vi "ocr subvi22.vi"(7 "char set file path":path, 9 "Manual ROI selection":bool, 10 "Image":T3) -> (1 "Read String":string, 3 "Image 2":T3(plugin-control))   [LabVIEW 2011]
uses:
  <vilib>/vision/NI_Vision_Development_Module.lvlib
  <vilib>/vision/Image Controls.llb/IMAQ Image.ctl
  <vilib>/vision/OCR.llb/IMAQ OCR Character Report 2.ctl
panel:
  out "subarray":i32[](array[numeric])
  out "Coordinates":i32[][](array[numeric])
  out "ROI Bounding Characters":T1 {"Contours"."Type" items=["No Selection", "Point", "Line", "Rectangle", "Oval", "Polygon", "Free", "Annulus", "Unused2", "Unused3", "Broken Line", "Free Hand Line", "Rotated Rectangle"]}
  out "Global Rectangle":i32[](array[numeric])
  out "Character Reports":T2[](array[typedef]) {"Character Statistics"."Threshold Range"."Upper value" format="%.2f"; "Character Statistics"."Threshold Range"."Lower value" format="%.2f"}
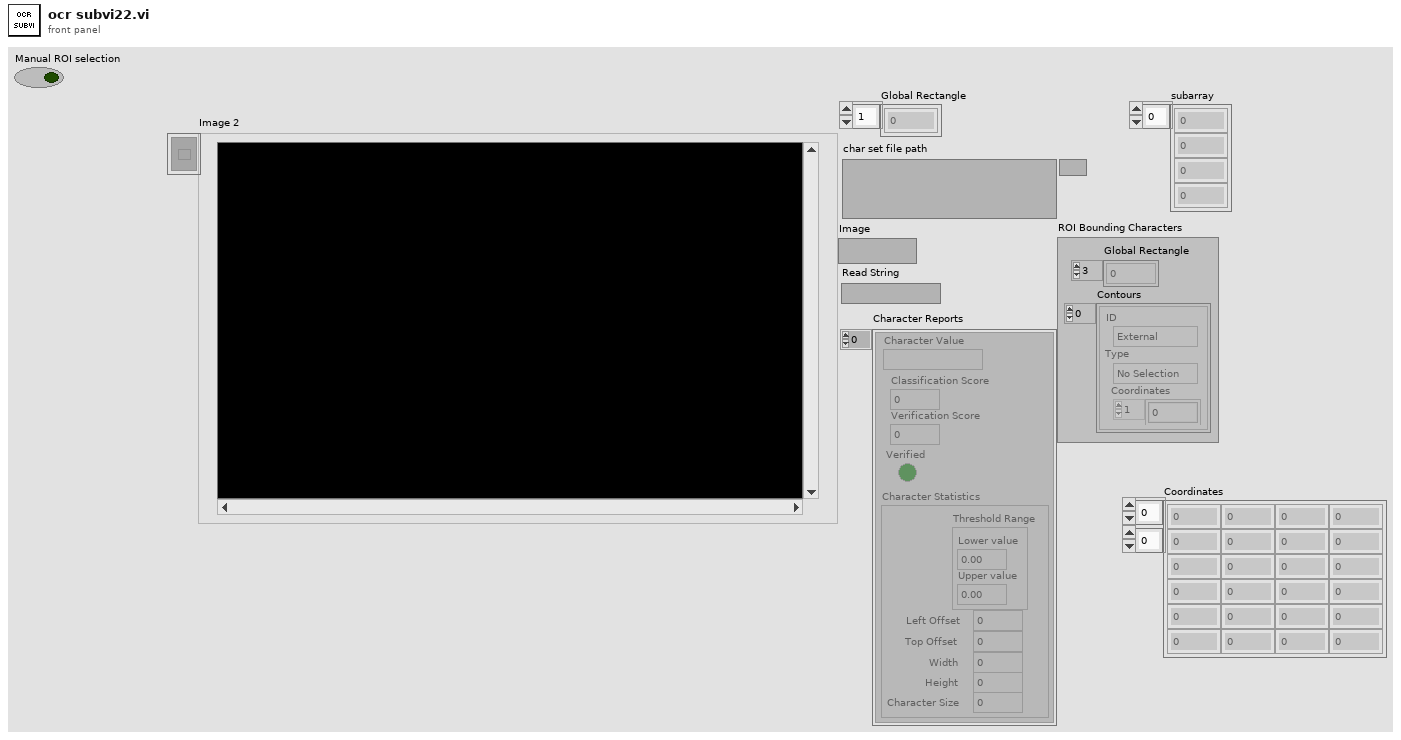
[diagram p1: front panel]
types:
  T1 = cluster{"Global Rectangle":i32[], "Contours":cluster{"ID":enum32{"External", "Internal"}, "Type":u32, "Coordinates":i32[]}[]}
  T2 = typedef "IMAQ OCR Character Report 2.ctl" = cluster{"Character Value":string, "Classification Score":i32, "Verification Score":i32, "Verified":bool, "Character Statistics":cluster{"Threshold Range":cluster{"Lower value":sgl, "Upper value":sgl}, "Left Offset":i32, "Top Offset":i32, "Width":i32, "Height":i32, "Character Size":i32}}
  T3 = typedef "IMAQ Image.ctl" = refnum<image>
  T4 = typedef "IMAQ OCR Session.ctl" = refnum<k1>
  T5 = cluster{i32[], cluster{"Contour Type":u32, "ROI Type":u32, i32[]}[]}
  T6 = cluster{"ID":enum32{"External", "Internal"}, "Type":u32, "Coordinates":i32[]}[]
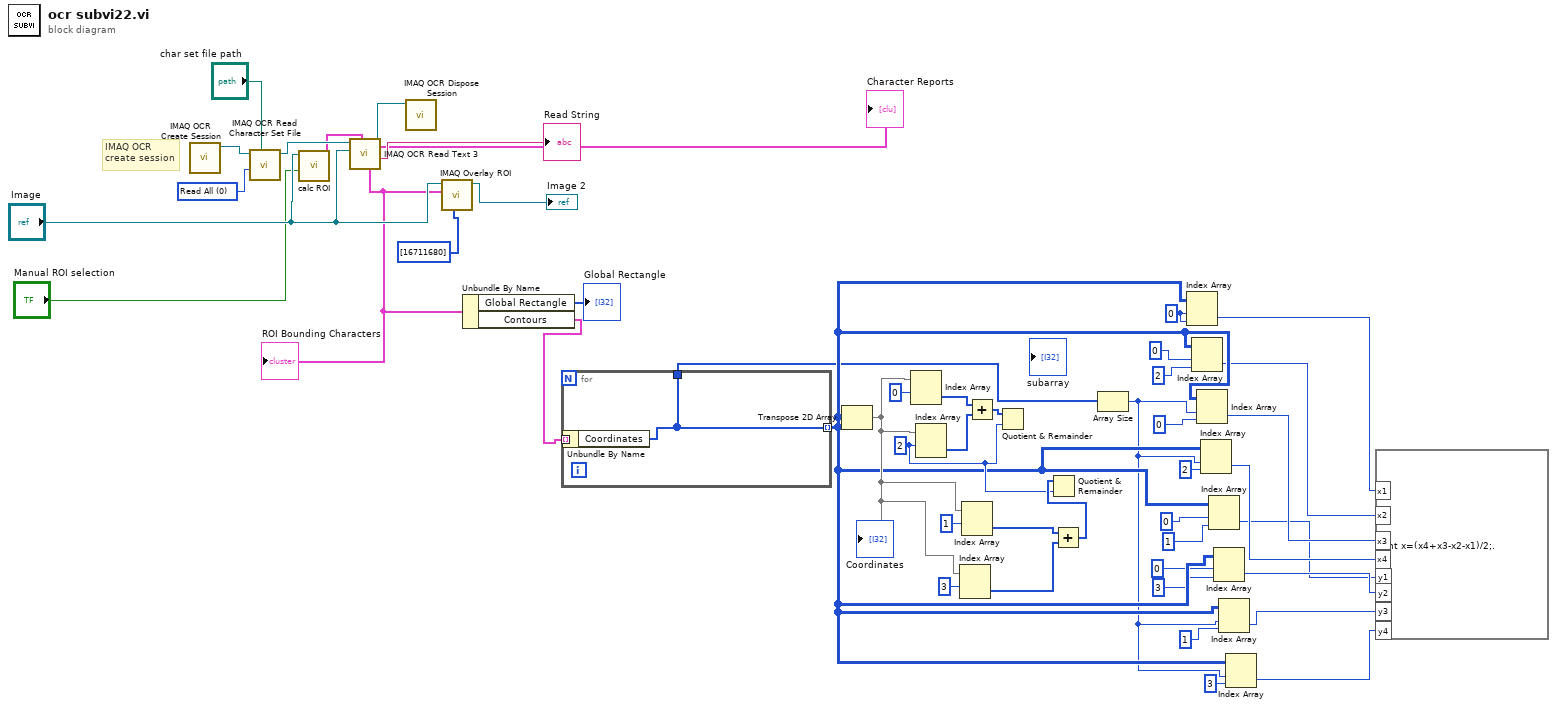
[diagram p0: block diagram]
diagram:
  w9 = 0 ("index (row)")
  w24 = 2 ("index")
  w48 = 0 items=["Read All", "Read Character Set Only", "Read Properties Only"] ("Read Options")
  # "IMAQ OCR \ncreate session"
  n1 = call "IMAQ OCR Create Session"() -> ("IMAQ OCR Session"=w47:T4)  [unwired: 1 in, 10 out]
  n2 = call "IMAQ OCR Read Character Set File"("File Path"="char set file path", "Read Options"=w48, "IMAQ OCR Session"=w47) -> ("IMAQ OCR Session (dup)"=w45:T4)  [unwired: 2 in, 6 out]
  n3 = call "calc ROI.vi"("Manual ROI selection"="Manual ROI selection", "Image"="Image") -> ("only ROI Cluster"=w43:T5)  [unwired: 9 in]
  n4 = call "IMAQ OCR Read Text 3"("ROI Descriptor"=w43, "Image"="Image", "IMAQ OCR Session"=w45) -> ("Read String"=→"Read String":string, "IMAQ OCR Session (dup)"=w40:T4, "ROI Bounding Characters"=w35:T1, "Character Reports"=→"Character Reports":T2[])  [unwired: 2 in, 3 out]
  "ROI Bounding Characters" <- w35
  n5 = call "IMAQ OCR Dispose Session"("IMAQ OCR Session"=w40) -> ()  [unwired: 1 in, 10 out]
  n6 = call "IMAQ Overlay ROI"("Colors (Green)"=u32[] [16711680], "ROI Descriptor"=w35, "Image"="Image") -> ("Image Out"=→"Image 2":T3)  [unwired: 3 in, 5 out]
  n7 = Unbundle By Name(w35) -> ("Global Rectangle"=→"Global Rectangle":i32[], "Contours"=w34:T6)
  n8 = for {
    tunnel: w34 -> [w50] mode=indexing
    tunnel: [w49] -> w18 mode=indexing
    tunnel: [w49] -> w17
    n9 = Unbundle By Name(w50) -> ("Coordinates"=w49:i32[])
  }
  n10 = Transpose 2D Array(2D array=w18) -> (transposed array=w23:i32[][])
  "Coordinates" <- w23
  n11 = Index Array(array=w23, index (row)=0 ("index")) -> (element=w30:i32[])  [unwired: 1 in]
  n12 = Index Array(array=w23, index (row)=w24) -> (element=w29:i32[])  [unwired: 1 in]
  n13 = Index Array(array=w23, index (row)=3 ("index")) -> (element=w27:i32[])  [unwired: 1 in]
  n14 = Index Array(array=w23, index (row)=1 ("index")) -> (element=w28:i32[])  [unwired: 1 in]
  n15 = Add(x=w30, y=w29) -> (x+y=w26:i32[])
  n16 = Quotient & Remainder(x=w26, y=w24) -> ()  [unwired: 2 out]
  n17 = Add(x=w28, y=w27) -> (x+y=w25:i32[])
  n18 = Quotient & Remainder(x=w25, y=w24) -> ()  [unwired: 2 out]
  n19 = Array Size(array=w17) -> (size(s)=w16:i32)
  n20 = Index Array(array=w18, index (row)=w9, index (col)=w9) -> (element=w8:i32)
  n21 = Index Array(array=w18, index (row)=0, index (col)=2 ("disabled index (col)")) -> (element=w7:i32)
  n22 = Index Array(array=w18, index (row)=w16, index (col)=0 ("disabled index (col)")) -> (element=w6:i32)
  n23 = Index Array(array=w18, index (row)=w16, index (col)=2 ("disabled index (col)")) -> (element=w5:i32)
  n24 = Index Array(array=w18, index (row)=0 ("disabled index (row)"), index (col)=1 ("disabled index (col)")) -> (element=w1:i32)
  n25 = Index Array(array=w18, index (row)=0 ("disabled index (row)"), index (col)=3 ("disabled index (col)")) -> (element=w2:i32)
  n26 = Index Array(array=w18, index (row)=w16, index (col)=1 ("disabled index (col)")) -> (element=w3:i32)
  n27 = Index Array(array=w18, index (row)=w16, index (col)=3 ("disabled index (col)")) -> (element=w4:i32)
  n28 = formula code="int x=(x4+x3-x2-x1)/2;."("x1"=w8, "x2"=w7, "x3"=w6, "x4"=w5, "y1"=w1, "y2"=w2, "y3"=w3, "y4"=w4) -> ()
